vi "test_simulated temperature waveform and scalar readings_mss.vi"(8 "Error In":errorcluster) -> (0 "Error Out":errorcluster)   [LabVIEW 2023]
uses:
  Measure and Stimulus Subsystems/Measure and Stimulus Subsystems.lvclass
panel:
  out "Powersensor Chart":waveform(dbl)(graph)
  in  "Stop":bool
  out "Photosensor Chart":dbl(graph)
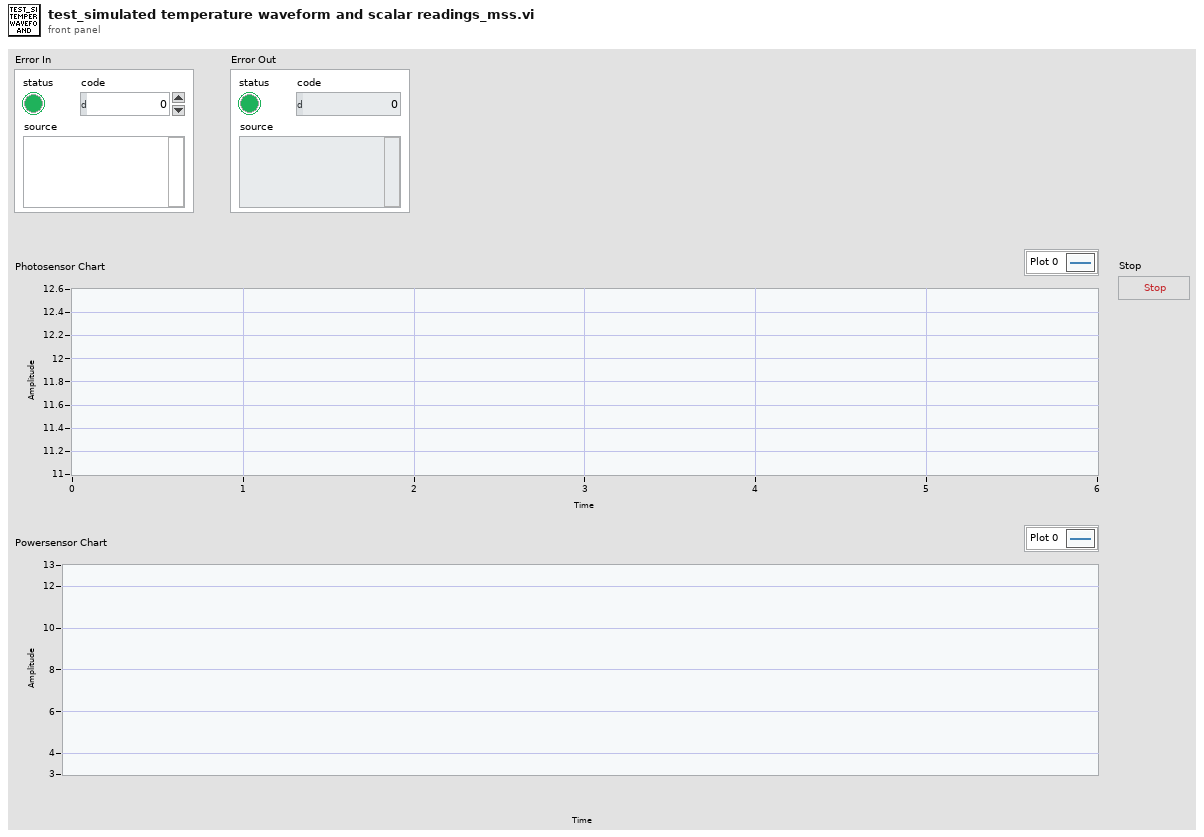
[diagram p1: front panel]
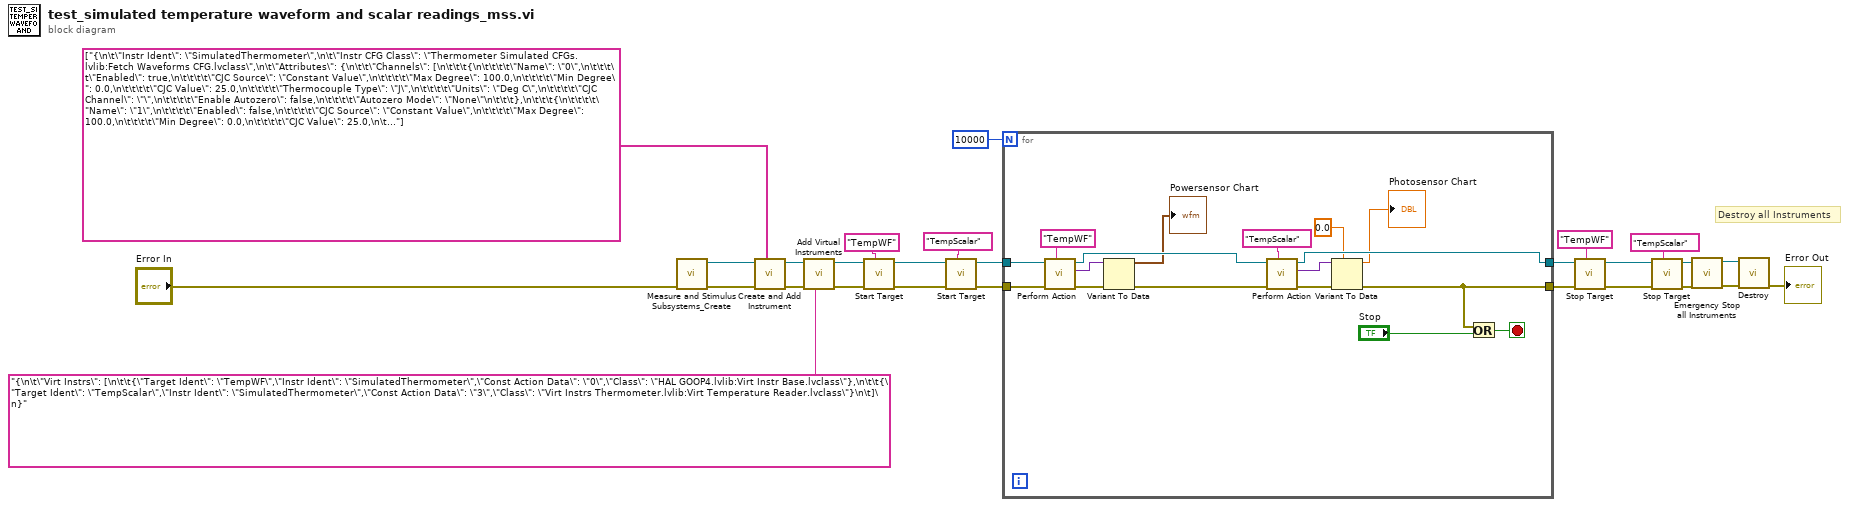
[diagram p0: block diagram]
diagram:
  # "Destroy all Instruments"
  n1 = call "Measure and Stimulus Subsystems_Create.vi"("Error In"="Error In") -> ("Error Out"=w26:errorcluster, "reference out"=w27:refnum<class "Measure and Stimulus Subsystems.lvclass">)  [unwired: 9 in]
  n2 = call "Create and Add Instrument.vi"("Physical Intr Configs"=string[] ["{\n\t\"Instr Ident\": \"SimulatedThermometer\",\n\t\"Instr CFG Class\": \"Thermometer Simulated CFGs.lvlib:Fetch Waveforms CFG.lvclass\",\n\t\"Attributes\": {\n\t\t\"Channels\": [\n\t\t\t{\n\t\t\t\t\"Name\": \"0\",\n\t\t\t\t\"Enabled\": true,\n\t\t\t\t\"CJC Source\": \"Constant Value\",\n\t\t\t\t\"Max Degree\": 100.0,\n\t\t\t\t\"Min Degree\": 0.0,\n\t\t\t\t\"CJC Value\": 25.0,\n\t\t\t\t\"Thermocouple Type\": \"J\",\n\t\t\t\t\"Units\": \"Deg C\",\n\t\t\t\t\"CJC Channel\": \"\",\n\t\t\t\t\"Enable Autozero\": false,\n\t\t\t\t\"Autozero Mode\": \"None\"\n\t\t\t},\n\t\t\t{\n\t\t\t\t\"Name\": \"1\",\n\t\t\t\t\"Enabled\": false,\n\t\t\t\t\"CJC Source\": \"Constant Value\",\n\t\t\t\t\"Max Degree\": 100.0,\n\t\t\t\t\"Min Degree\": 0.0,\n\t\t\t\t\"CJC Value\": 25.0,\n\t\t\t\t\"Thermocouple Type\": \"J\",\n\t\t\t\t\"Units\": \"Deg C\",\n\t\t\t\t\"CJC Channel\": \"\",\n\t\t\t\t\"Enable Autozero\": false,\n\t\t\t\t\"Autozero Mode\": \"None\"\n\t\t\t},\n\t\t\t{\n\t\t\t\t\"Name\": \"2\",\n\t\t\t\t\"Enabled\": false,\n\t\t\t\t\"CJC Source\": \"Constant Value\",\n\t\t\t\t\"Max Degree\": 100.0,\n\t\t\t\t\"Min Degree\": 0.0,\n\t\t\t\t\"CJC Value\": 25.0,\n\t\t\t\t\"Thermocouple Type\": \"J\",\n\t\t\t\t\"Units\": \"Deg C\",\n\t\t\t\t\"CJC Channel\": \"\",\n\t\t\t\t\"Enable Autozero\": false,\n\t\t\t\t\"Autozero Mode\": \"None\"\n\t\t\t},\n\t\t\t{\n\t\t\t\t\"Name\": \"3\",\n\t\t\t\t\"Enabled\": true,\n\t\t\t\t\"CJC Source\": \"Constant Value\",\n\t\t\t\t\"Max Degree\": 100.0,\n\t\t\t\t\"Min Degree\": 0.0,\n\t\t\t\t\"CJC Value\": 25.0,\n\t\t\t\t\"Thermocouple Type\": \"J\",\n\t\t\t\t\"Units\": \"Deg C\",\n\t\t\t\t\"CJC Channel\": \"\",\n\t\t\t\t\"Enable Autozero\": false,\n\t\t\t\t\"Autozero Mode\": \"None\"\n\t\t\t}\n\t ],\n\t\t\t\"Timing\": {\n\t\t\t\"Samples per Channel\": 1000,\n\t\t\t\"Sample Mode\": \"Continuous Samples\",\n\t\t\t\"Sample Rate\": 20.0,\n\t\t\t\"Sample Clock Source\": \"OnboardClock\",\n\t\t\t\"Active Edge\": \"Rising\"\n\t\t},\n\t\t\"Trigger\": {\n\t\t\t\"Trigger Type\": \"No Trigger\"\n\t\t},\n\t\t\"Acquisition\": {\n\t\t\t\"Relative To\": \"Current Read Position\",\n\t\t\t\"Overwrite\": \"Do Not Overwrite Unread Samples\",\n\t\t\t\"Samples per Fetch\": -1,\n\t\t\t\"Timeout\": 1.0\n\t\t}\n\t}\n}"], "Error In"=w26, "reference in"=w27) -> ("Error Out"=w20:errorcluster, "reference out"=w3:refnum<class "Measure and Stimulus Subsystems.lvclass">)  [unwired: 7 in]
  n3 = call "Add Virtual Instruments.vi"("<JSON CFG>"="{\n\t\"Virt Instrs\": [\n\t\t{\"Target Ident\": \"TempWF\",\"Instr Ident\": \"SimulatedThermometer\",\"Const Action Data\": \"0\",\"Class\": \"HAL GOOP4.lvlib:Virt Instr Base.lvclass\"},\n\t\t{\"Target Ident\": \"TempScalar\",\"Instr Ident\": \"SimulatedThermometer\",\"Const Action Data\": \"3\",\"Class\": \"Virt Instrs Thermometer.lvlib:Virt Temperature Reader.lvclass\"}\n\t]\n}", "Error In"=w20, "reference in"=w3) -> ("Error Out"=w4:errorcluster, "reference out"=w2:refnum<class "Measure and Stimulus Subsystems.lvclass">)  [unwired: 7 in]
  n4 = call "Start Target.vi"("Target Ident"="TempWF", "Error In"=w4, "reference in"=w2) -> ("Error Out"=w18:errorcluster, "reference out"=w16:refnum<class "Measure and Stimulus Subsystems.lvclass">)  [unwired: 7 in]
  n5 = call "Start Target.vi"("Target Ident"="TempScalar", "Error In"=w18, "reference in"=w16) -> ("Error Out"=w17:errorcluster, "reference out"=w15:refnum<class "Measure and Stimulus Subsystems.lvclass">)  [unwired: 7 in]
  n6 = for {
    N: 10000 -> [_]
    tunnel: w17 -> [w37]
    tunnel: w15 -> [w36]
    tunnel: [w38] -> w11
    tunnel: [w40] -> w24
    stop <- w44 stop-if-true
    n7 = call "Perform Action.vi"("Target Ident"="TempWF" ("Target Identifier"), "Error In"=w37, "reference in"=w36) -> ("Error Out"=w35:errorcluster, "Output"=w31:variant, "reference out"=w32:refnum<class "Measure and Stimulus Subsystems.lvclass">)  [unwired: 6 in]
    n8 = Variant To Data(error in=w35, Variant=w31) -> (data=→"Powersensor Chart":waveform(dbl), error out=w33:errorcluster)  [unwired: 1 in]
    n9 = call "Perform Action.vi"("Target Ident"="TempScalar" ("Target Identifier"), "Error In"=w33, "reference in"=w32) -> ("Error Out"=w42:errorcluster, "Output"=w39:variant, "reference out"=w38:refnum<class "Measure and Stimulus Subsystems.lvclass">)  [unwired: 6 in]
    n10 = Variant To Data(error in=w42, type=0.0, Variant=w39) -> (data=→"Photosensor Chart":dbl, error out=w40:errorcluster)
    n11 = Or(x=w40, y="Stop") -> (x .or. y?=w44:bool)
  }
  n12 = call "Stop Target.vi"("Target Ident"="TempWF", "Error In"=w24, "reference in"=w11) -> ("Error Out"=w12:errorcluster, "reference out"=w9:refnum<class "Measure and Stimulus Subsystems.lvclass">)  [unwired: 7 in]
  n13 = call "Stop Target.vi"("Target Ident"="TempScalar", "Error In"=w12, "reference in"=w9) -> ("Error Out"=w10:errorcluster, "reference out"=w8:refnum<class "Measure and Stimulus Subsystems.lvclass">)  [unwired: 7 in]
  n14 = call "Emergency Stop all Instruments.vi"("Error In"=w10, "reference in"=w8) -> ("Error Out"=w23:errorcluster, "reference out"=w22:refnum<class "Measure and Stimulus Subsystems.lvclass">)  [unwired: 8 in]
  n15 = call "Destroy.vi"("Error In"=w23, "reference in"=w22) -> ("Error Out"=→"Error Out":errorcluster)  [unwired: 8 in, 1 out]
